vi "Close.vi"(8 "error in":errorcluster, 11 "OnOff Channels in":refnum<class "OnOff Channels.lvclass">) -> (0 "error out":errorcluster, 3 "OnOff Channels out":refnum<class "OnOff Channels.lvclass">)   [LabVIEW 2023, in "OnOff Channels.lvclass"]
uses:
  OnOff Channels.lvclass
  OnOff Channels.lvclass/OnOff Channels.ctl
  <vilib>/ADAS Replay HIL/AdasHilServices/AdasHilServices Fill In Error Info Ex.vi
  <vilib>/ADAS Replay HIL/AdasHilServices/AdasHilChannelServices.lvlib
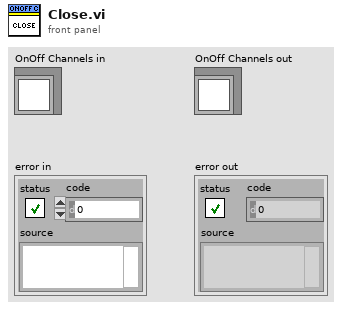
[diagram p1: front panel]
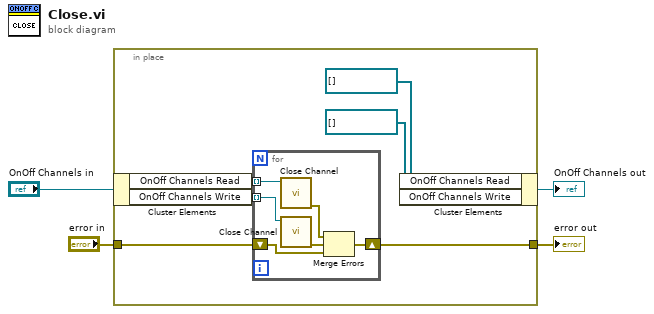
[diagram p0: block diagram]
diagram:
  n1 = in-place {
    in-place-border: "error in" -> [w10]
    in-place-border: [w9] -> w1
    n2 = in-place-cluster #1("OnOff Channels in") -> ("OnOff Channels Read"=w8:refnum<k21>[], "OnOff Channels Write"=w7:refnum<k21>[])
    n3 = for {
      tunnel: w8 -> [w16] mode=indexing
      tunnel: w7 -> [w15] mode=indexing
      shift-right: [w14] -> w9
      shift-left: w10 -> [w11]
      n4 = call <vilib>:"Close Channel.vi"("ADAS HIL Channel"=w16) -> ("error out"=w13:errorcluster)  [unwired: 10 in]
      n5 = call <vilib>:"Close Channel.vi"("ADAS HIL Channel"=w15) -> ("error out"=w12:errorcluster)  [unwired: 10 in]
      n6 = Merge Errors(w13, w12, w11) -> (w14:errorcluster)
    }
    n7 = in-place-cluster #1("OnOff Channels Read"=refnum<k21>[] [] ("Control Mode Read"), "OnOff Channels Write"=refnum<k21>[] [] ("Control Mode Read")) -> (→"OnOff Channels out":refnum<class "OnOff Channels.lvclass">)
  }
  "error out" <- w1
